vi "Master Setup GetPath(pla).vi"(10 "path in":path=path "C:/Revolutionary Engineering/Setup Files/Default/Shop Cell 3/~ETC ECCS Setup Files 06-21-2010 08 56 AM.ect") -> (2 "path array":path[](array[path]))   [LabVIEW 2017]
doc: "Get the path from the *.pla"
uses:
  Playback PC/Playback Setup.ctl
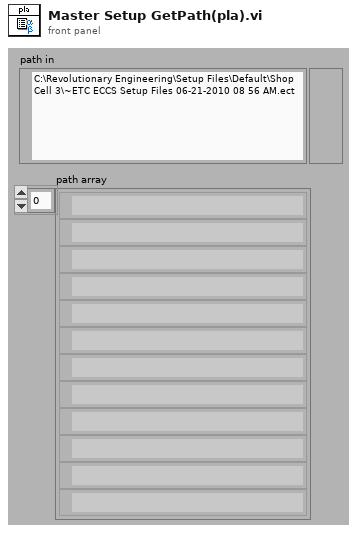
[diagram p1: front panel]
types:
  T1 = enum16{"open", "replace", "create", "open or create", "replace or create", "replace or create with confirmation"}
  T2 = typedef "Playback Setup.ctl" = cluster{"File Path":path, "Excel Worksheet":dbl, "Label Row":dbl, "Unit Label Row":dbl, "Data Start Row":dbl, "Data End Row":dbl}
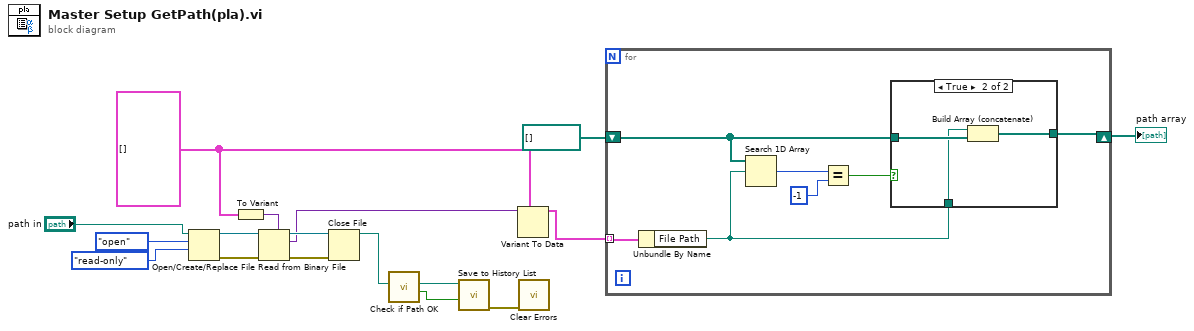
[diagram p0: block diagram]
diagram:
  w17 = T2[] [] ("Playback Setup")
  n1 = Open/Create/Replace File(file path (use dialog)="path in", operation (0:open)=T1."open", access (0:read/write)=enum16{"read/write", "read-only", "write-only"}."read-only") -> (refnum out=w10:refnum<file>, error out=w11:errorcluster)  [unwired: 3 in, 1 out]
  n2 = To Variant(anything=w17) -> (Variant=w13:variant)
  n3 = Read from Binary File(5:w13, 8:w11, 11:w10) -> (0:w9:errorcluster, 2:w2:variant, 3:w8:refnum<file>)  [unwired: 4 out]
  n4 = Close File(refnum=w8, error in=w9) -> (path=w5:path)  [unwired: 1 out]
  n5 = call "Check if Path OK.vi"("Path"=w5) -> ("Path OK"=w6:bool, "Path"=w4:path)  [unwired: 8 in, 1 out]
  n6 = call "Save to History List.vi"("Write to History File"=w6, "File Path In"=w4) -> ("error out"=w3:errorcluster)  [unwired: 6 in, 3 out]
  n7 = Variant To Data(type=w17, Variant=w2) -> (data=w14:T2[])  [unwired: 1 in, 1 out]
  n8 = call <vilib>:"Clear Errors.vi"("error in (no error)"=w3) -> ()  [unwired: 5 in, 2 out]
  n9 = for {
    tunnel: w14 -> [w24] mode=indexing
    shift-right: [w23] -> w15
    shift-left: path[] [] -> [w22]
    n10 = Unbundle By Name(w24) -> ("File Path"=w21:path)
    n11 = Search 1D Array(1D array=w22, element=w21) -> (index of element=w20:i32)  [unwired: 1 in]
    n12 = Equal?(x=w20, y=-1) -> (x = y?=w18:bool)
    n13 = case shown="True" w18 {
      tunnel: [w25 w28] -> w23
      tunnel: w22 -> [w25 w27]
      tunnel: w21 -> [_ w26]
      frame False {
      }
      frame True {
        n14 = Build Array (concatenate)(w26, w27) -> (w28:path[])
      }
    }
  }
  "path array" <- w15
